vi "Log_MessageHandler_CreateNewLogFileName.vi"(8 "error in (no error)":errorcluster, 11 "MessageHandler in":refnum<class "MessageHandler.lvclass">) -> (0 "error out":errorcluster, 3 "MessageHandler out":refnum<class "MessageHandler.lvclass">)   [LabVIEW 2013, in "MessageHandler.lvclass"]
uses:
  MessageHandler.lvclass
  MessageHandler.lvclass/MessageHandler.ctl
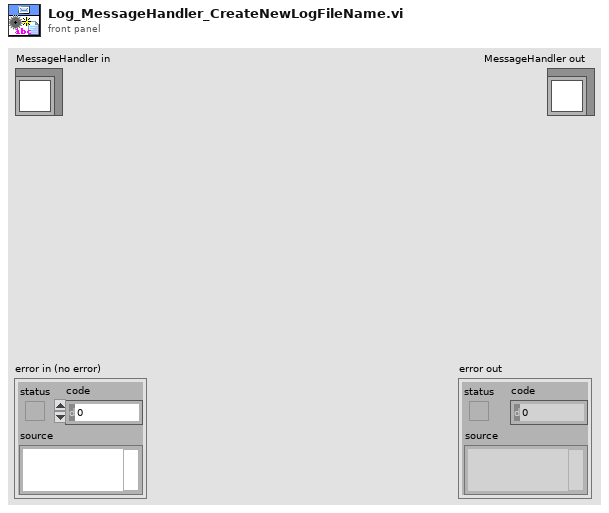
[diagram p1: front panel]
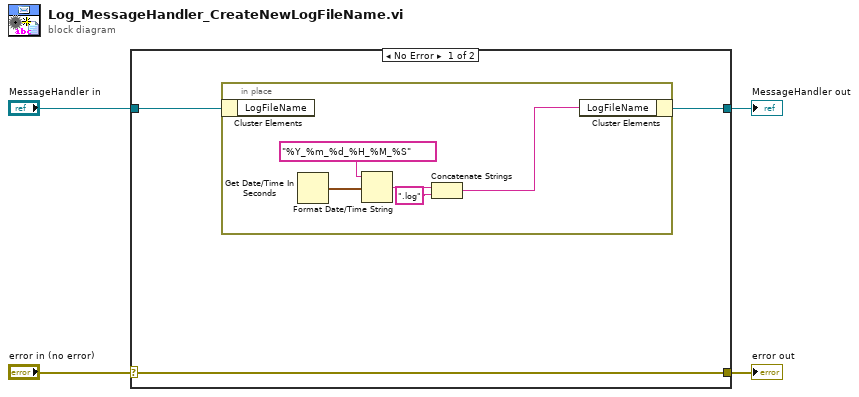
[diagram p0: block diagram]
diagram:
  n1 = case shown="No Error" "error in (no error)" {
    selector: "error in (no error)" -> [w7 w14]
    tunnel: [w7 w14] -> w3
    tunnel: [w5 w13] -> w1
    tunnel: "MessageHandler in" -> [w6 w13]
    frame No Error {
      n2 = in-place {
        n3 = in-place-cluster #1(w6) -> ()  [unwired: 1 out]
        n4 = Get Date/Time In Seconds() -> (seconds since 1Jan1904=w9:timestamp)
        n5 = Format Date/Time String(time format string (%c)="%Y_%m_%d_%H_%M_%S", seconds (now)=w9) -> (date/time string=w11:string)  [unwired: 1 in]
        n6 = Concatenate Strings(w11, ".log" ("string")) -> (w8:string)
        n7 = in-place-cluster #1("LogFileName"=w8) -> (w5:refnum<class "MessageHandler.lvclass">)
      }
    }
    frame Error {
    }
  }
  "error out" <- w3
  "MessageHandler out" <- w1
